vi "generate header.vi"(11 "data in":u32[](array[numeric])) -> (3 "data + header":u32[](array[numeric]))   [LabVIEW 2013]
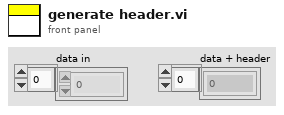
[diagram p1: front panel]
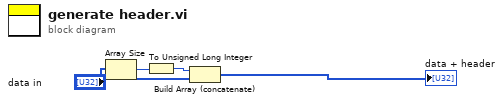
[diagram p0: block diagram]
diagram:
  n1 = Array Size(array="data in") -> (size(s)=w2:i32)
  n2 = To Unsigned Long Integer(number=w2) -> (unsigned 32bit integer=w3:u32)
  n3 = Build Array (concatenate)(w3, "data in") -> (→"data + header":u32[])
